vi "cms123.vi"() -> ()   [LabVIEW 2015]
uses:
  <vilib>/NXT/Block Support/NXT_InputPort.ctl
  <vilib>/NXT/Block Support/NXT_OutputPort.ctl
  <vilib>/NXT/Dual Mode Library/Sensors/Light_On.vi
  <vilib>/NXT/NXTIO Xnodes/NXTIONodeSubVIs/NXTMoveMotors.vi
  <vilib>/NXT/Dual Mode Library/Waits/Wait_Num.vi
  <vilib>/NXT/Dual Mode Library/Motors/Rotation.vi
  <vilib>/NXT/Subs/LVHSConnector.ctl
  <vilib>/NXT/NXTIO Xnodes/AddressXNode/NXTIOAddress.xnode
  <vilib>/NXT/NXTIO Xnodes/NXTIOXNode/NXTIO.xnode
  <vilib>/NXT/LegoClasses/BrickReference/BrickReference.lvclass
panel:
  in  "stop":bool
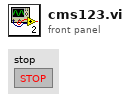
[diagram p1: front panel]
types:
  T1 = typedef "NXT_OutputPort.ctl" = u8
  T2 = typedef "NXT_InputPort.ctl" = u32
  T3 = typedef "LVHSConnector.ctl" = refnum<class "BrickReference.lvclass">
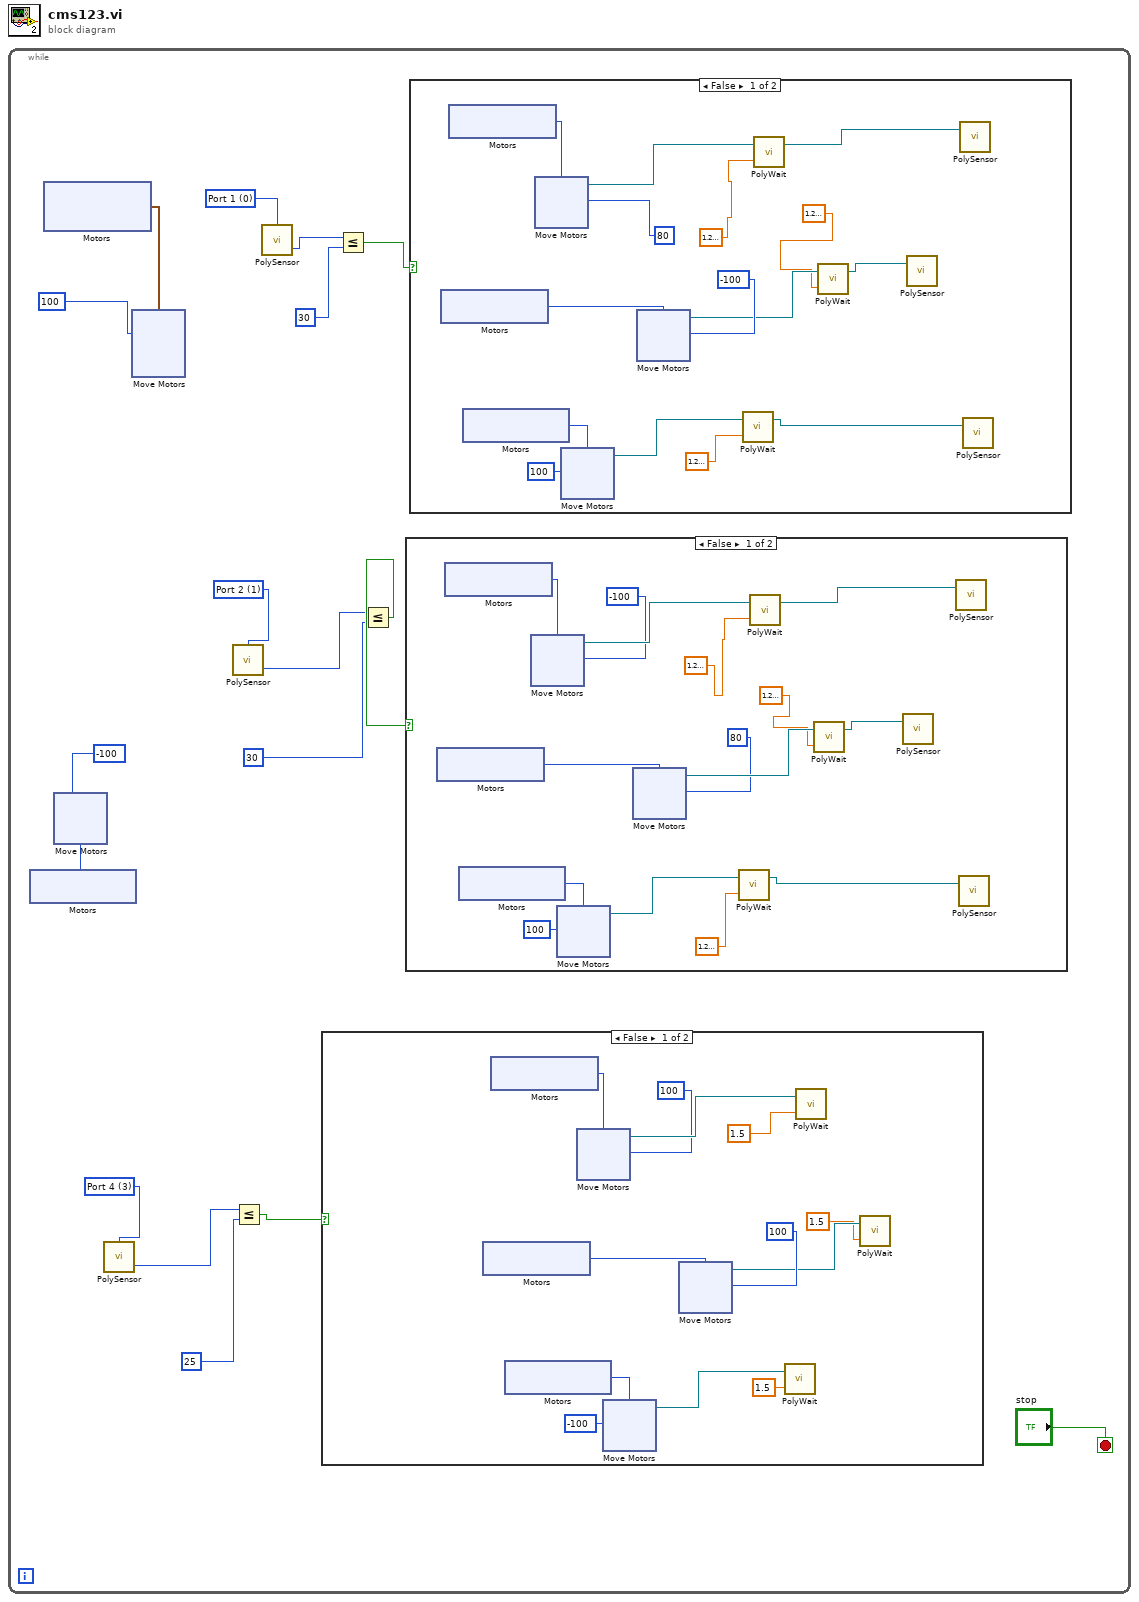
[diagram p0: block diagram]
diagram:
  n1 = while {
    stop <- "stop" stop-if-true
    w4 = T2 3 items=["Port 1", "Port 2", "Port 3", "Port 4"] ("Port (Port 3)")
    w8 = T2 0 items=["Port 1", "Port 2", "Port 3", "Port 4"] ("Port (Port 3)")
    w11 = T2 1 items=["Port 1", "Port 2", "Port 3", "Port 4"] ("Port (Port 3)")
    n2 = xnode "Motors"() -> ("Motor"=w13:T1)
    n3 = xnode "Motors"() -> ("Motor"=w14:cluster{"Port":T1, "Port":T1})
    n4 = xnode "Move Motors"("Power/Speed 1"=i8 -100, "Motors"=w13) -> ()  [unwired: 1 in, 1 out]
    n5 = call-poly <vilib>:"PolySensor.vi"("Port (Port 3)"=w4) -> ("Scaled Value"=w3:i16)  [unwired: 2 in, 1 out]
    n6 = xnode "Move Motors"("Power/Speed 1"=i8 100, "Motors"=w14) -> ()  [unwired: 2 in, 1 out]
    n7 = call-poly <vilib>:"PolySensor.vi"("Port (Port 3)"=w11) -> ("Scaled Value"=w10:i16)  [unwired: 2 in, 1 out]
    n8 = Less Or Equal?(x=w3, y=i16 25) -> (x <= y?=w1:bool)
    n9 = call-poly <vilib>:"PolySensor.vi"("Port (Port 3)"=w8) -> ("Scaled Value"=w7:i16)  [unwired: 2 in, 1 out]
    n10 = case shown="False" w1 {
      frame False {
        n11 = xnode "Motors"() -> ("Motor"=w22:T1)
        n12 = xnode "Motors"() -> ("Motor"=w29:T1)
        n13 = xnode "Motors"() -> ("Motor"=w28:T1)
        n14 = xnode "Move Motors"("Power/Speed 1"=i16 100 ("y"), "Motors"=w29) -> ("NXT/EV3"=w24:T3)  [unwired: 1 in]
        n15 = xnode "Move Motors"("Power/Speed 1"=i8 -100, "Motors"=w28) -> ("NXT/EV3"=w23:T3)  [unwired: 1 in]
        n16 = xnode "Move Motors"("Power/Speed 1"=i16 100 ("y"), "Motors"=w22) -> ("NXT/EV3"=w20:T3)  [unwired: 1 in]
        n17 = call-poly <vilib>:"PolyWait.vi"("Time (1 sec)"=sgl 1.5, "NXT/EV3"=w23) -> ()  [unwired: 2 in, 1 out]
        n18 = call-poly <vilib>:"PolyWait.vi"("Time (1 sec)"=sgl 1.5, "NXT/EV3"=w24) -> ()  [unwired: 2 in, 1 out]
        n19 = call-poly <vilib>:"PolyWait.vi"("Time (1 sec)"=sgl 1.5, "NXT/EV3"=w20) -> ()  [unwired: 2 in, 1 out]
      }
      frame True {
      }
    }
    n20 = Less Or Equal?(x=w7, y=i16 30) -> (x <= y?=w5:bool)
    n21 = Less Or Equal?(x=w10, y=i16 30) -> (x <= y?=w12:bool)
    n22 = case shown="False" w12 {
      frame False {
        n23 = xnode "Motors"() -> ("Motor"=w100:T1)
        n24 = xnode "Motors"() -> ("Motor"=w107:T1)
        n25 = xnode "Motors"() -> ("Motor"=w106:T1)
        n26 = xnode "Move Motors"("Power/Speed 1"=i16 -100 ("y"), "Motors"=w107) -> ("NXT/EV3"=w104:T3)  [unwired: 1 in]
        n27 = xnode "Move Motors"("Power/Speed 1"=i8 100, "Motors"=w106) -> ("NXT/EV3"=w103:T3)  [unwired: 1 in]
        n28 = xnode "Move Motors"("Power/Speed 1"=i16 80 ("y"), "Motors"=w100) -> ("NXT/EV3"=w99:T3)  [unwired: 1 in]
        n29 = call-poly <vilib>:"PolyWait.vi"("Time (1 sec)"=sgl 1.3, "NXT/EV3"=w103) -> ("NXT/EV3"=w101:T3)  [unwired: 2 in]
        n30 = call-poly <vilib>:"PolyWait.vi"("Time (1 sec)"=sgl 1.3, "NXT/EV3"=w104) -> ("NXT/EV3"=w102:T3)  [unwired: 2 in]
        n31 = call-poly <vilib>:"PolyWait.vi"("Time (1 sec)"=sgl 1.3, "NXT/EV3"=w99) -> ("NXT/EV3"=w97:T3)  [unwired: 2 in]
        n32 = call-poly <vilib>:"PolySensor.vi"("NXT/EV3"=w97) -> ()  [unwired: 2 in, 2 out]
        n33 = call-poly <vilib>:"PolySensor.vi"("NXT/EV3"=w102) -> ()  [unwired: 2 in, 2 out]
        n34 = call-poly <vilib>:"PolySensor.vi"("NXT/EV3"=w101) -> ()  [unwired: 2 in, 2 out]
      }
      frame True {
      }
    }
    n35 = case shown="False" w5 {
      frame False {
        n36 = xnode "Motors"() -> ("Motor"=w61:T1)
        n37 = xnode "Motors"() -> ("Motor"=w68:T1)
        n38 = xnode "Motors"() -> ("Motor"=w67:T1)
        n39 = xnode "Move Motors"("Power/Speed 1"=i16 80 ("y"), "Motors"=w68) -> ("NXT/EV3"=w65:T3)  [unwired: 1 in]
        n40 = xnode "Move Motors"("Power/Speed 1"=i8 100, "Motors"=w67) -> ("NXT/EV3"=w64:T3)  [unwired: 1 in]
        n41 = xnode "Move Motors"("Power/Speed 1"=i16 -100 ("y"), "Motors"=w61) -> ("NXT/EV3"=w59:T3)  [unwired: 1 in]
        n42 = call-poly <vilib>:"PolyWait.vi"("Time (1 sec)"=sgl 1.3, "NXT/EV3"=w64) -> ("NXT/EV3"=w62:T3)  [unwired: 2 in]
        n43 = call-poly <vilib>:"PolyWait.vi"("Time (1 sec)"=sgl 1.3, "NXT/EV3"=w65) -> ("NXT/EV3"=w63:T3)  [unwired: 2 in]
        n44 = call-poly <vilib>:"PolyWait.vi"("Time (1 sec)"=sgl 1.3, "NXT/EV3"=w59) -> ("NXT/EV3"=w57:T3)  [unwired: 2 in]
        n45 = call-poly <vilib>:"PolySensor.vi"("NXT/EV3"=w57) -> ()  [unwired: 2 in, 2 out]
        n46 = call-poly <vilib>:"PolySensor.vi"("NXT/EV3"=w63) -> ()  [unwired: 2 in, 2 out]
        n47 = call-poly <vilib>:"PolySensor.vi"("NXT/EV3"=w62) -> ()  [unwired: 2 in, 2 out]
      }
      frame True {
      }
    }
  }
